vi "Init LUTs.vi"(8 "error in":errorcluster, 11 "object in":refnum<class "SDS1000 Base CFG.lvclass">) -> (0 "error out":errorcluster, 3 "object out":refnum<class "SDS1000 Base CFG.lvclass">)   [LabVIEW 2023, in "OWON SDS1022.lvlib" / "SDS1000 Base CFG.lvclass"]
uses:
  SDS1000 Base CFG.lvclass
  SDS1000 Base CFG.lvclass/SDS1000 Base CFG.ctl
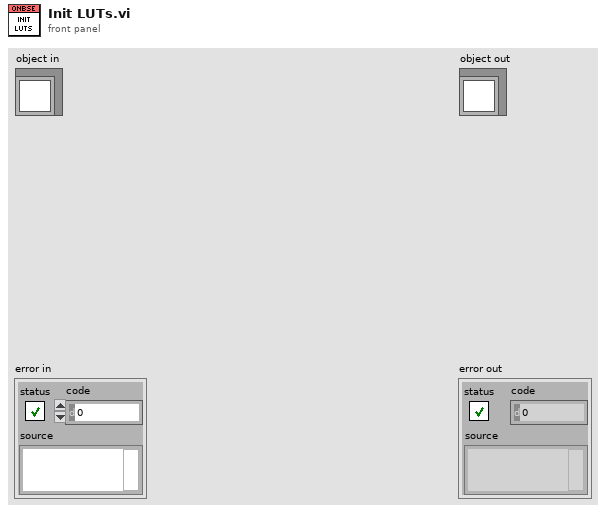
[diagram p1: front panel]
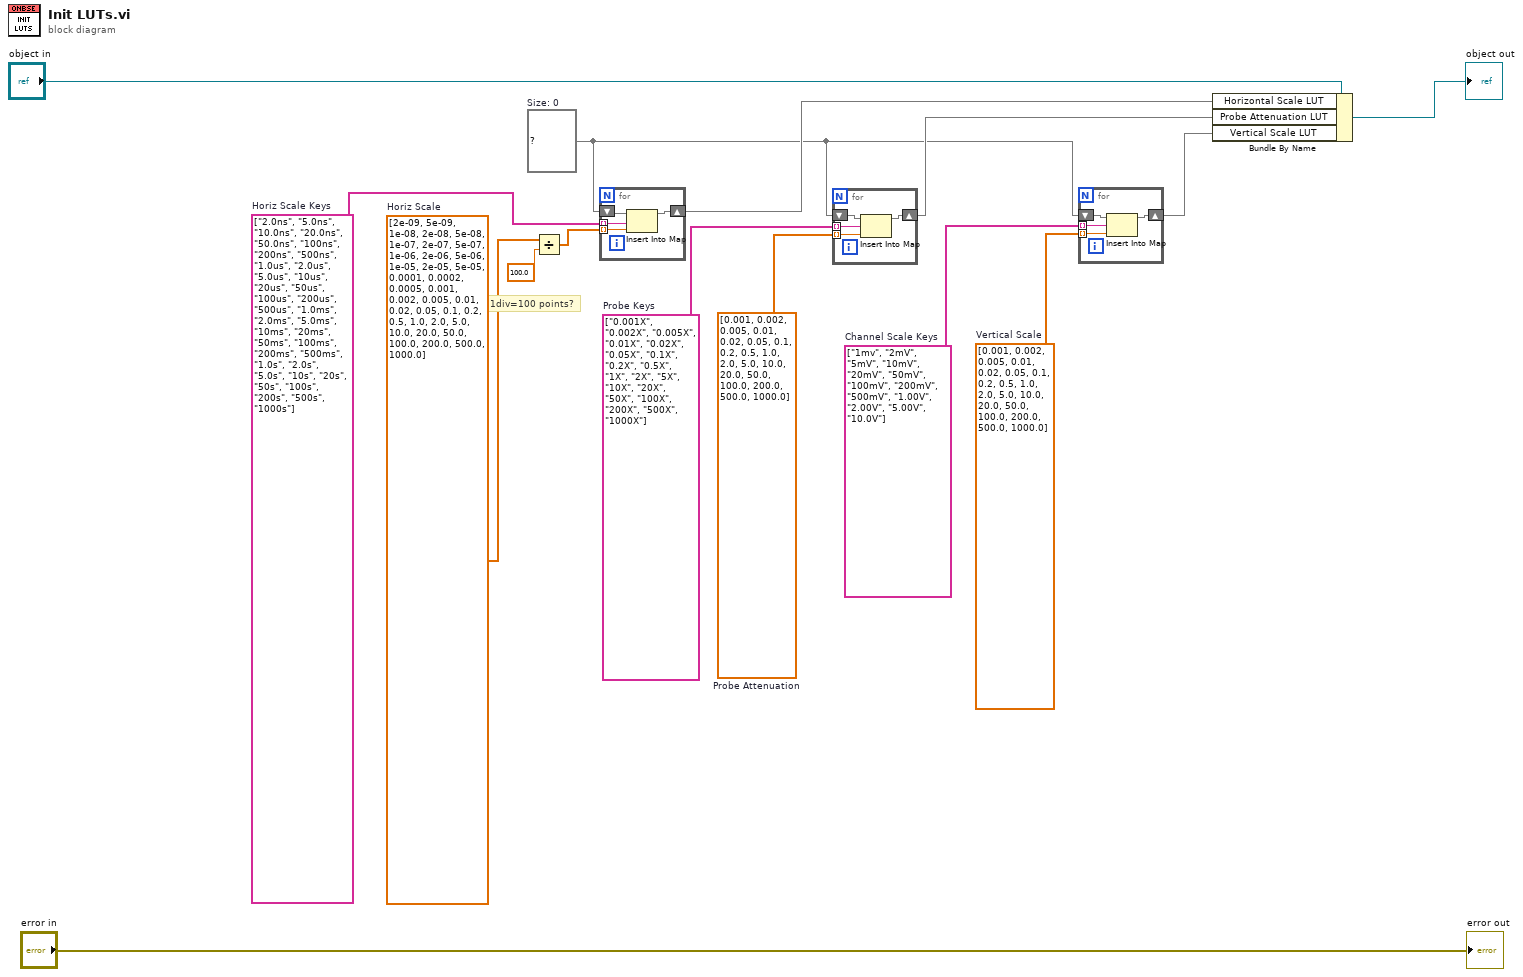
[diagram p0: block diagram]
diagram:
  w1 = map{string, dbl} {}  # Size: 0
  w4 = dbl[] [0.001, 0.002, 0.005, 0.01, 0.02, 0.05, 0.1, 0.2, 0.5, 1.0, 2.0, 5.0, 10.0, 20.0, 50.0, 100.0, 200.0, 500.0, 1000.0]  # Vertical Scale
  w7 = dbl[] [0.001, 0.002, 0.005, 0.01, 0.02, 0.05, 0.1, 0.2, 0.5, 1.0, 2.0, 5.0, 10.0, 20.0, 50.0, 100.0, 200.0, 500.0, 1000.0]  # Probe Attenuation
  w8 = string[] ["0.001X", "0.002X", "0.005X", "0.01X", "0.02X", "0.05X", "0.1X", "0.2X", "0.5X", "1X", "2X", "5X", "10X", "20X", "50X", "100X", "200X", "500X", "1000X"]  # Probe Keys
  w5 = string[] ["1mv", "2mV", "5mV", "10mV", "20mV", "50mV", "100mV", "200mV", "500mV", "1.00V", "2.00V", "5.00V", "10.0V"]  # Channel Scale Keys
  w10 = dbl[] [2e-09, 5e-09, 1e-08, 2e-08, 5e-08, 1e-07, 2e-07, 5e-07, 1e-06, 2e-06, 5e-06, 1e-05, 2e-05, 5e-05, 0.0001, 0.0002, 0.0005, 0.001, 0.002, 0.005, 0.01, 0.02, 0.05, 0.1, 0.2, 0.5, 1.0, 2.0, 5.0, 10.0, 20.0, 50.0, 100.0, 200.0, 500.0, 1000.0]  # Horiz Scale
  w12 = string[] ["2.0ns", "5.0ns", "10.0ns", "20.0ns", "50.0ns", "100ns", "200ns", "500ns", "1.0us", "2.0us", "5.0us", "10us", "20us", "50us", "100us", "200us", "500us", "1.0ms", "2.0ms", "5.0ms", "10ms", "20ms", "50ms", "100ms", "200ms", "500ms", "1.0s", "2.0s", "5.0s", "10s", "20s", "50s", "100s", "200s", "500s", "1000s"]  # Horiz Scale Keys
  # "1div=100 points?"
  n1 = Divide(x=w10, y=100.0) -> (x/y=w9:dbl[])
  n2 = for {
    shift-right: [w18] -> w2
    shift-left: w1 -> [w19]
    tunnel: w12 -> [w17] mode=indexing
    tunnel: w9 -> [w16] mode=indexing
    n3 = Insert Into Map(map in=w19, key=w17, value=w16) -> (map out=w18:map{string, dbl})  [unwired: 2 out]
  }
  n4 = for {
    tunnel: w8 -> [w22] mode=indexing
    tunnel: w7 -> [w23] mode=indexing
    shift-right: [w20] -> w6
    shift-left: w1 -> [w21]
    n5 = Insert Into Map(map in=w21, key=w22, value=w23) -> (map out=w20:map{string, dbl})  [unwired: 2 out]
  }
  n6 = for {
    tunnel: w5 -> [w26] mode=indexing
    tunnel: w4 -> [w27] mode=indexing
    shift-right: [w24] -> w3
    shift-left: w1 -> [w25]
    n7 = Insert Into Map(map in=w25, key=w26, value=w27) -> (map out=w24:map{string, dbl})  [unwired: 2 out]
  }
  n8 = Bundle By Name(cluster="object in", "Horizontal Scale LUT"=w2, "Probe Attenuation LUT"=w6, "Vertical Scale LUT"=w3) -> (→"object out":refnum<class "SDS1000 Base CFG.lvclass">)
  "error out" <- "error in"
